vi "Read Number of Channels.vi"(8 "error in (no error)":errorcluster, 11 "Mag Lab Digitizer in":refnum<class "Mag Lab Digitizer.lvclass">) -> (0 "error out":errorcluster, 2 "Number of Channels":i32, 3 "Mag Lab Digitizer out":refnum<class "Mag Lab Digitizer.lvclass">)   [LabVIEW 2015, in "Mag Lab Digitizer.lvclass"]
uses:
  Mag Lab Digitizer.lvclass
  Mag Lab Digitizer.lvclass/Mag Lab Digitizer.ctl
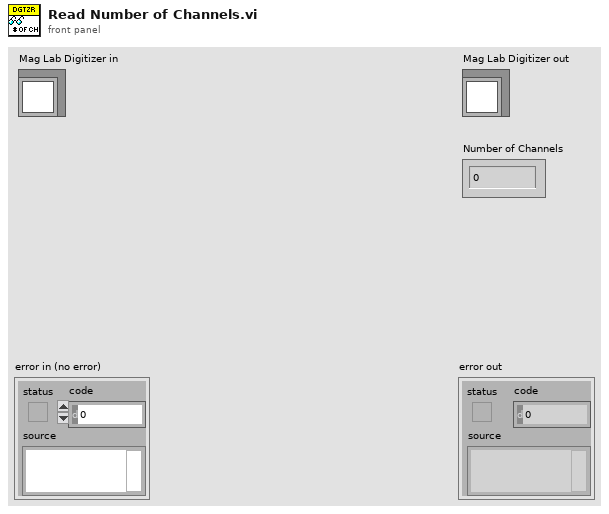
[diagram p1: front panel]
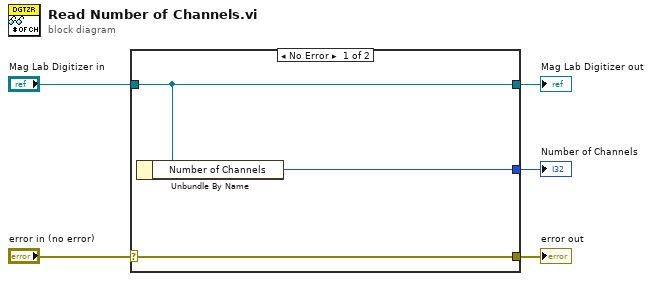
[diagram p0: block diagram]
diagram:
  n1 = case shown="No Error" "error in (no error)" {
    selector: "error in (no error)" -> [w8 w9]
    tunnel: [w8 w9] -> w4
    tunnel: [w7 w10] -> w2
    tunnel: "Mag Lab Digitizer in" -> [w7 w10]
    tunnel: [w6 _] -> w1
    frame No Error {
      n2 = Unbundle By Name(w7) -> ("Number of Channels"=w6:i32)
    }
    frame Error {
    }
  }
  "error out" <- w4
  "Mag Lab Digitizer out" <- w2
  "Number of Channels" <- w1
